vi "Write kickX.vi"(8 "error in (no error)":errorcluster, 10 "kickX":dbl, 11 "KickToSkill_v2 in":refnum<class "KickToSkill_v2.lvclass">) -> (0 "error out":errorcluster, 3 "KickToSkill_v2 out":refnum<class "KickToSkill_v2.lvclass">)   [LabVIEW 2023, in "KickToSkill_v2.lvclass"]
uses:
  KickToSkill_v2.lvclass
  KickToSkill_v2.lvclass/KickToSkill_v2.ctl
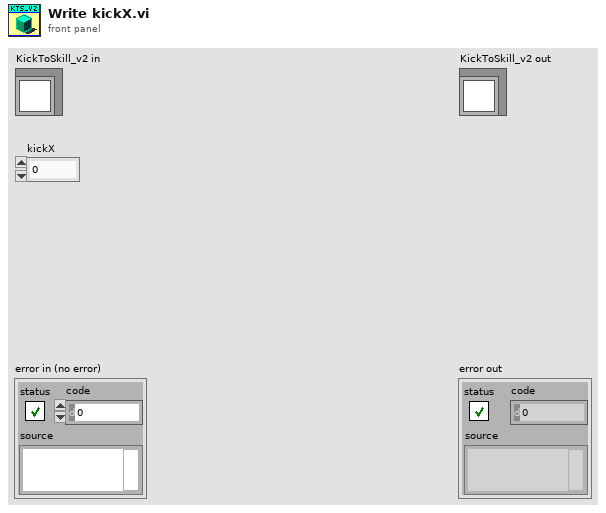
[diagram p1: front panel]
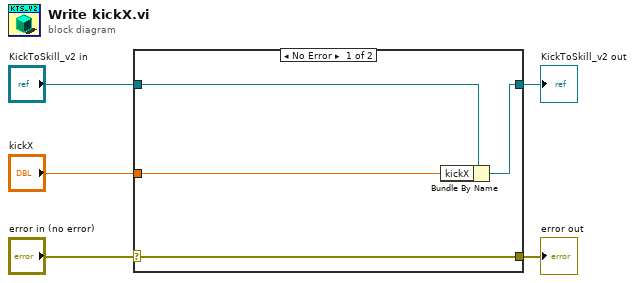
[diagram p0: block diagram]
diagram:
  n1 = case shown="No Error" "error in (no error)" {
    selector: "error in (no error)" -> [w9 w10]
    tunnel: [w9 w10] -> w4
    tunnel: [w7 w11] -> w2
    tunnel: "KickToSkill_v2 in" -> [w8 w11]
    tunnel: "kickX" -> [w6 _]
    frame No Error {
      n2 = Bundle By Name(cluster=w8, "kickX"=w6) -> (w7:refnum<class "KickToSkill_v2.lvclass">)
    }
    frame Error {
    }
  }
  "error out" <- w4
  "KickToSkill_v2 out" <- w2
